vi "ESCAPES_Main.vi"() -> ()   [LabVIEW 2018]
panel:
  in  "Tab Control":enum32{"Main", "Files", "Setup", "Tools"}(tab)
  out "Rep":i32
  in  "Participant Code":string="ESCAPES_"
  out "Time":string
  in  "Filename":string
  in  "Log Data Button":bool
  in  "Add Pcode":bool
  out "Participant ID":string
  in  "View Saved Data":bool
  in  "Recorded Data":i32(listbox)
  in  "Webcam Enable?":bool=TRUE
  in  "VISA resource name":refnum<visa-resource-name>="COM16"
  in  "Serial Settings":T1={"baud rate"=115200, "data bits"=8, "parity"=enum."None", "stop bits"=10, "flow control"=0} {"flow control" items=["None"=0, "XON/XOFF"=1, "RTS/CTS"=2, "DTR/DSR"=4]; "stop bits" items=["1.0"=10, "1.5"=15, "2.0"=20]; "data bits" min=5 max=8 step=1; "baud rate" items=["75"=75, "110"=110, "134"=134, "150"=150, "300"=300, "600"=600, "1200"=1200, "1800"=1800, "2400"=2400, "4800"=4800, "7200"=7200, "9600"=9600, "14400"=14400, "19200"=19200, "28800"=28800, "38400"=38400, "56000"=56000, "57600"=57600, "115200"=115200, "128000"=128000, "230400"=230400]}
  in  "Stop webcam":bool
  in  "Test Webcam":bool
  in  "Retrieve Data Button":bool
  in  "Stream Button":bool
  out "Data Path":path
  # "scapes"
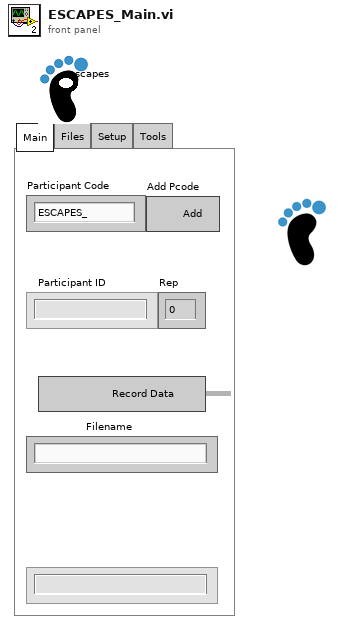
[diagram p1: front panel]
types:
  T1 = cluster{"baud rate":u32, "data bits":u16, "parity":enum16{"None", "Odd", "Even", "Mark", "Space"}, "stop bits":u16, "flow control":u16}
  T2 = enum16{"Record to File", "Preview 320x240", "Preview 640x480"}
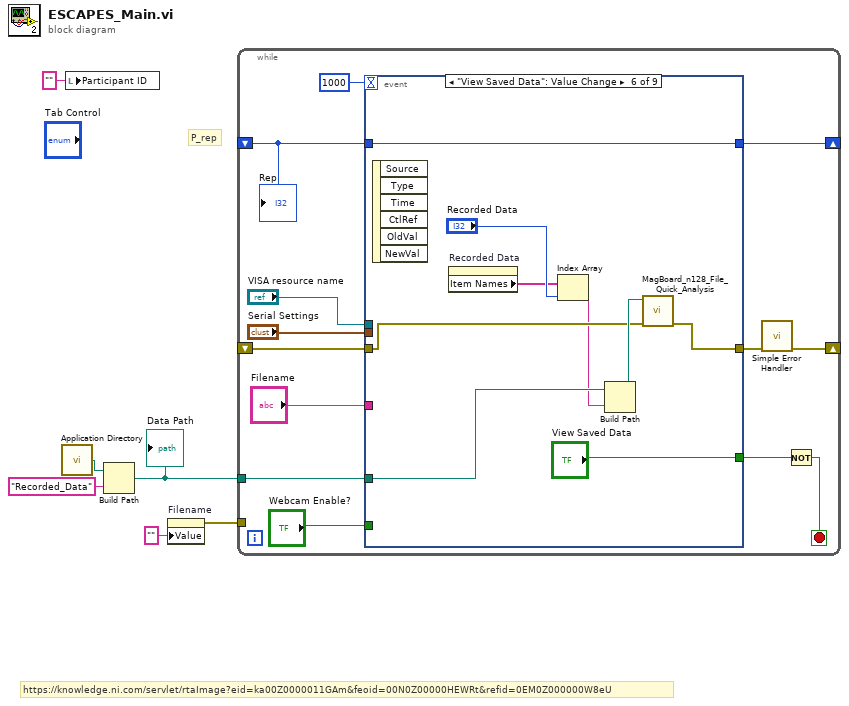
[diagram p0: block diagram]
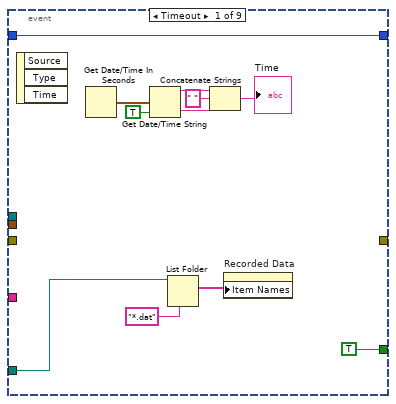
[diagram p2: hidden frame]
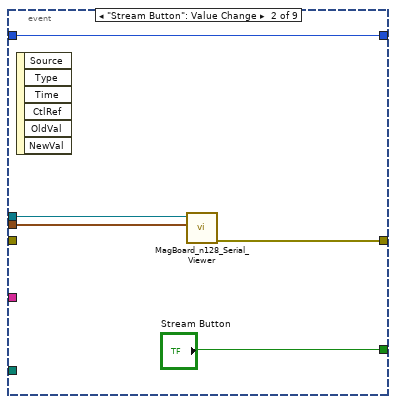
[diagram p3: hidden frame]
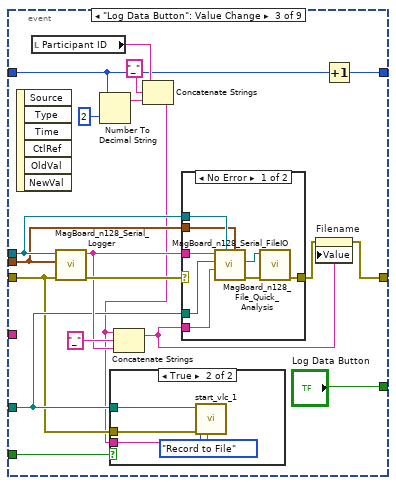
[diagram p4: hidden frame]
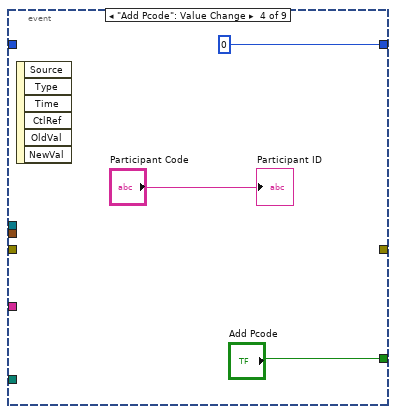
[diagram p7: hidden frame]
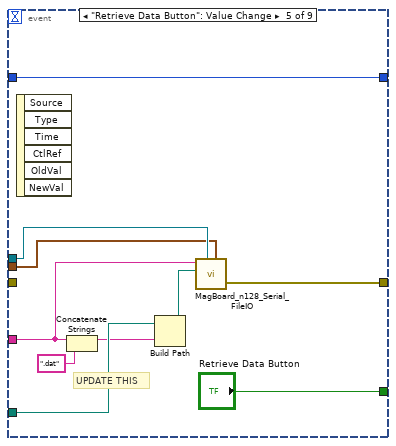
[diagram p8: hidden frame]
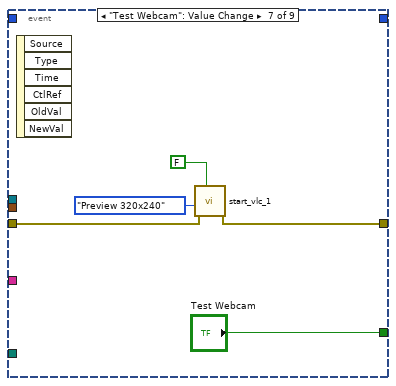
[diagram p9: hidden frame]
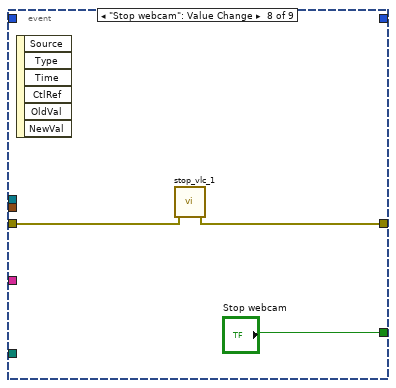
[diagram p10: hidden frame]
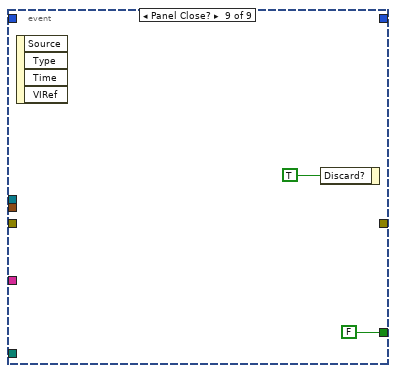
[diagram p11: hidden frame]
diagram:
  # "https://knowledge.ni.com/servlet/rtaImage?eid=ka00Z0000011GAm&feoid=00N0Z00000HEWRt&refid=0EM0Z000000W8eU"
  # "P_rep"
  n1 = call <vilib>:"Application Directory.vi"() -> ("Application Directory"=w4:path)
  n2 = local write "Participant ID"("" ("Participant ID")) -> ()
  n3 = Build Path(base path=w4, name or relative path="Recorded_Data" ("string")) -> (appended path=w2:path)
  "Data Path" <- w2
  n4 = property on="Filename" class="Str"("Value"="" ("Filename")) -> (error out=w3:errorcluster)  [unwired: 2 in, 1 out]
  n5 = while {
    shift-right: [w11] -> _
    shift-left: _ -> [w14]
    tunnel: w2 -> [w13]
    tunnel: w3 -> [_]
    shift-right: [w9] -> _
    shift-left: _ -> [w8]
    stop <- w18 stop-if-true
    n6 = event shown="[5] \"View Saved Data\": Value Change" {
      selector: _ -> [_ _ _ _ _ _ _ _ _]
      dyn-events: _ -> [_ _ _ _ _ _ _ _ _]
      timeout: 1000 -> [_ _ _ _ _ _ _ _ _]
      tunnel: [TRUE ("Stream Button") "Stream Button" "Log Data Button" "Add Pcode" "Retrieve Data Button" "View Saved Data" "Test Webcam" "Stop webcam" FALSE ("Stream Button")] -> w19
      tunnel: "VISA resource name" -> [_ w34 w51 _ w73 _ _ _ _]
      tunnel: "Serial Settings" -> [_ w33 w50 _ w72 _ _ _ _]
      tunnel: [_ w32 w54 _ w74 w85 w90 w95 _] -> w12
      tunnel: "Filename" -> [_ _ _ _ w77 _ _ _ _]
      tunnel: w14 -> [_ _ w38 _ _ w84 w91 w96 _]
      tunnel: w13 -> [w29 _ w40 _ w78 w88 _ _ _]
      tunnel: w8 -> [w21 w31 w41 _ w71 w87 _ _ _]
      tunnel: [w21 w31 w42 0 w71 w87 _ _ _] -> w9
      tunnel: "Webcam Enable?" -> [_ _ w39 _ _ _ _ _ _]
      event Timeout {
        n7 = event-data() -> ()  [unwired: 1 in, 3 out]
        n8 = Get Date/Time In Seconds() -> (seconds since 1Jan1904=w28:timestamp)
        n9 = Get Date/Time String(seconds (now)=w28, want seconds? (F)=TRUE) -> (date string=w24:string, time string=w25:string)  [unwired: 1 in]
        n10 = List Folder(path=w29, pattern="*.dat") -> (filenames=w20:string[])  [unwired: 2 in, 3 out]
        n11 = Concatenate Strings(w24, " " ("string"), w25) -> (→"Time":string)
        n12 = property on="Recorded Data" class="LstBox (strict)"("Item Names"=w20) -> ()  [unwired: 2 in, 2 out]
      }
      event "Stream Button": Value Change {
        n13 = event-data() -> ()  [unwired: 1 in, 6 out]
        n14 = call "MagBoard_n128_Serial_Viewer.vi"("Serial Settings"=w33, "VISA resource name"=w34) -> ("error out"=w32:errorcluster)  [unwired: 9 in]
      }
      event "Log Data Button": Value Change {
        n15 = event-data() -> ()  [unwired: 1 in, 6 out]
        n16 = local read "Participant ID"() -> (w45:string)
        n17 = call "MagBoard_n128_Serial_Logger.vi"("error in (no error)"=w38, "Serial Settings"=w50, "VISA resource name"=w51) -> ("error out"=w52:errorcluster, "Filename"=w47:string)  [unwired: 7 in]
        n18 = Number To Decimal String(number=w41, width (-)=i16 2) -> (decimal integer string=w43:string)
        n19 = Concatenate Strings(w45, "_" ("Filename"), w43) -> (w36:string)
        n20 = case shown="True" w39 {
          tunnel: w38 -> [_ w58]
          tunnel: w36 -> [_ w57]
          tunnel: w40 -> [_ w56]
          frame False {
          }
          frame True {
            n21 = call "start_vlc_1.vi"("Filename"=w57, "error in (no error)"=w58, "Operation"=T2."Record to File", "video_capture_dir"=w56) -> ()  [unwired: 5 in, 3 out]
          }
        }
        n22 = Concatenate Strings(w36, "_" ("Filename"), w47) -> (w37:string)
        n23 = case shown="No Error" w52 {
          selector: w52 -> [_ w67]
          tunnel: w51 -> [w66 _]
          tunnel: w50 -> [w65 _]
          tunnel: w47 -> [w64 _]
          tunnel: w37 -> [w60 _]
          tunnel: [w62 w67] -> w49
          tunnel: w40 -> [w59 _]
          frame No Error {
            n24 = call "MagBoard_n128_Serial_FileIO.vi"("Serial Settings"=w65, "VISA resource name"=w66, "File_Code"=w60, "Directory"=w59, "Remote Filename"=w64) -> ("error out"=w63:errorcluster, "FilePath Out"=w61:path)  [unwired: 4 in, 1 out]
            n25 = call "MagBoard_n128_File_Quick_Analysis.vi"("error in"=w63, "Path"=w61) -> ("error out"=w62:errorcluster)  [unwired: 9 in]
          }
          frame Error {
          }
        }
        n26 = property on="Filename" class="Str"(error in=w49, "Value"=w37) -> (error out=w54:errorcluster)  [unwired: 1 in, 1 out]
        n27 = Increment(x=w41) -> (x+1=w42:i32)
      }
      event "Add Pcode": Value Change {
        n28 = event-data() -> ()  [unwired: 1 in, 6 out]
        "Participant ID" <- "Participant Code"
      }
      event "Retrieve Data Button": Value Change {
        # "UPDATE THIS"
        n29 = event-data() -> ()  [unwired: 1 in, 6 out]
        n30 = Concatenate Strings(w77, ".dat" ("Filename")) -> (w76:string)
        n31 = Build Path(base path=w78, name or relative path=w76) -> (appended path=w79:path)
        n32 = call "MagBoard_n128_Serial_FileIO.vi"("Serial Settings"=w72, "VISA resource name"=w73, "Directory"=w79, "Remote Filename"=w77) -> ("error out"=w74:errorcluster)  [unwired: 5 in, 2 out]
      }
      event "View Saved Data": Value Change {
        n33 = event-data() -> ()  [unwired: 1 in, 6 out]
        n34 = property on="Recorded Data" class="LstBox (strict)"() -> ("Item Names"=w82:string[])  [unwired: 2 in, 2 out]
        n35 = Index Array(array=w82, index="Recorded Data") -> (element=w81:string)
        n36 = Build Path(base path=w88, name or relative path=w81) -> (appended path=w86:path)
        n37 = call "MagBoard_n128_File_Quick_Analysis.vi"("error in"=w84, "Path"=w86) -> ("error out"=w85:errorcluster)  [unwired: 9 in]
      }
      event "Test Webcam": Value Change {
        n38 = event-data() -> ()  [unwired: 1 in, 6 out]
        n39 = call "start_vlc_1.vi"("wait until completion? (F)"=FALSE ("wait until completion? (T)"), "error in (no error)"=w91, "Operation"=T2."Preview 320x240") -> ("error out"=w90:errorcluster)  [unwired: 6 in, 2 out]
      }
      event "Stop webcam": Value Change {
        n40 = event-data() -> ()  [unwired: 1 in, 6 out]
        n41 = call "stop_vlc_1.vi"("error in (no error)"=w96) -> ("error out"=w95:errorcluster)  [unwired: 10 in]
      }
      event Panel Close? {
        n42 = event-data() -> ()  [unwired: 1 in, 4 out]
        n43 = event-data("Discard?"=TRUE) -> ()  [unwired: 1 in, 1 out]
      }
    }
    n44 = call <vilib>:"Simple Error Handler.vi"("error in (no error)"=w12) -> ("error out"=w11:errorcluster)  [unwired: 4 in, 4 out]
    n45 = Not(x=w19) -> (.not. x?=w18:bool)
    "Rep" <- w8
  }
